vi "LowLevelController.vi"(4 "Left Lin Vel 2":dbl, 5 "Power Left":bool, 6 "Right Lin Vel 2":dbl, 7 "Power Right":bool, 8 "Right Lin Vel":dbl, 9 "Ref Velocity":dbl, 10 "Turn U":dbl, 11 "Left Lin Vel":dbl) -> ()   [LabVIEW 2017]
uses:
  MotorCommands.vi
  FrictionCompensatedU.vi
  <vilib>/Simulation/Implementation/Shared/SIMSCR Execution Mode.ctl
  <vilib>/Simulation/Scripting/Companion Diagram/SimConfigNode/SimParams.ctl
  <vilib>/Simulation/Scripting/Companion Diagram/SimConfigNode/_simSolvers.ctl
  <vilib>/Simulation/Param Hierarchy/Typedefs/SIMPH Param Control Actions.ctl
  <vilib>/Simulation/Implementation/Shared/NILVSim_ParamChanged.vi
  <vilib>/Simulation/Implementation/Shared/NILVSIM_BeginStep.vi
  <vilib>/Simulation/SignalArithmetic/Implementation/NILVSim Gain.llb/SIM Gain (scalar).vi
  <vilib>/Simulation/DiscreteLinear/Implementation/NILVSim Discrete Integrator Direct.llb/SIM Discrete Integrator Backward-Trap (scalar).vi
  <vilib>/Simulation/Implementation/Shared/NILVSim_Manager.vi
  <vilib>/Utility/error.llb/Clear Errors.vi
  <vilib>/Simulation/Implementation/Shared/NILVSim_FinalizeModel.vi
  <vilib>/Simulation/Implementation/Shared/SIM Unbundle Sim Info.vi
  <vilib>/Simulation/Implementation/Shared/SIMSH Read Queue.vi
  <vilib>/Simulation/Implementation/Shared/NILVSim_Initialize.vi
  <vilib>/Simulation/Utility/Implementation/NILVSim Get Time and IsAcceptedStep.vi
  <vilib>/Simulation/Implementation/Shared/NILVSim_GetModelError.vi
  <vilib>/Simulation/Implementation/Shared/SIM SimErrorHandler.vi
  <vilib>/Simulation/Implementation/Shared/SIM Bundle Sim Info.vi
  <vilib>/Simulation/Scripting/Companion Diagram/SimConfigNode/SimDog.xnode
  <vilib>/Simulation/Implementation/XNodeFramework/SimXNode/SimX.xnode
  <vilib>/Simulation/Implementation/Shared/NI_SIM_Implementation.lvlib
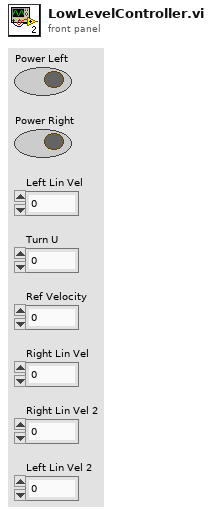
[diagram p1: front panel]
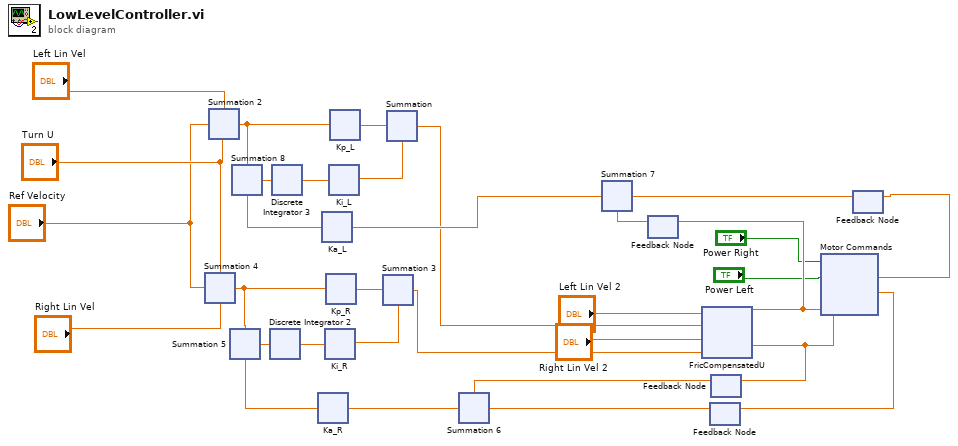
[diagram p0: block diagram]
diagram:
  n1 = xnode ("Summation 4")("Operand1"="Turn U", "Operand2"="Ref Velocity", "Operand3"="Right Lin Vel") -> ("Result"=w17:dbl)
  n2 = xnode ("Summation 2")("Operand1"="Left Lin Vel", "Operand2"="Ref Velocity", "Operand3"="Turn U") -> ("Result"=w30:dbl)
  n3 = xnode "Kp_R"("input"=w17) -> ("output"=w9:dbl)  [unwired: 3 in]
  n4 = xnode "Kp_L"("input"=w30) -> ("output"=w5:dbl)  [unwired: 3 in]
  n5 = feedback #1 ("Feedback Node 3")() -> (w27:dbl)  [unwired: 1 in]
  n6 = feedback #2 ("Feedback Node 2")() -> (w22:dbl)  [unwired: 1 in]
  n7 = feedback #3() -> (w23:dbl)  [unwired: 1 in]
  n8 = xnode ("Summation 6")("Operand1"=w23, "Operand2"=w22) -> ("Result"=w19:dbl)
  n9 = xnode "Ka_R"("input"=w19) -> ("output"=w18:dbl)  [unwired: 3 in]
  n10 = xnode ("Summation 5")("Operand1"=w17, "Operand2"=w18) -> ("Result"=w16:dbl)
  n11 = xnode ("Discrete Integrator 2")("input"=w16) -> ("output"=w8:dbl)  [unwired: 11 in, 1 out]
  n12 = xnode "Ki_R"("input"=w8) -> ("output"=w14:dbl)  [unwired: 3 in]
  n13 = xnode ("Summation 3")("Operand1"=w9, "Operand2"=w14) -> ("Result"=w11:dbl)
  n14 = feedback #4 ("Feedback Node 4")() -> (w25:dbl)  [unwired: 1 in]
  n15 = xnode ("Summation 7")("Operand1"=w25, "Operand2"=w27) -> ("Result"=w24:dbl)
  n16 = xnode "Ka_L"("input"=w24) -> ("output"=w31:dbl)  [unwired: 3 in]
  n17 = xnode ("Summation 8")("Operand1"=w30, "Operand2"=w31) -> ("Result"=w29:dbl)
  n18 = xnode ("Discrete Integrator 3")("input"=w29) -> ("output"=w15:dbl)  [unwired: 11 in, 1 out]
  n19 = xnode "Ki_L"("input"=w15) -> ("output"=w6:dbl)  [unwired: 3 in]
  n20 = xnode ("Summation")("Operand1"=w5, "Operand2"=w6) -> ("Result"=w12:dbl)
  n21 = xnode "FricCompensatedU"("u_Right"=w11, "Right Lin Vel"="Right Lin Vel 2", "u_Left"=w12, "Left Lin Vel"="Left Lin Vel 2") -> ("RightU"=w20:dbl, "LeftU"=w26:dbl)
  n22 = feedback-in #1 ("4")(w26) -> ()
  n23 = feedback-in #3 ("2")(w20) -> ()
  n24 = xnode "Motor Commands"("u_L"=w26, "u_R"=w20, "Power Left"="Power Left", "Power Right"="Power Right") -> ("satU_R"=w21:dbl, "satU_L"=w28:dbl)  [unwired: 6 out]
  n25 = feedback-in #2 ("3")(w21) -> ()
  n26 = feedback-in #4 ("5")(w28) -> ()
